vi "Gather Test Data - Heatup Test.vi"(0 "Agilent Scan List":string="101,102,103,104,105,106,107,108,109,110,111,112,113,114,115,116", 1 "Semiphore":T3, 2 "Equipment":T5={"COM Port"="COM1", "MW100"="MW100", "AG34970"="A-34972A", "Chamber"="WT500"}, 5 "Tank Display Ref":refnum<vi>, 7 "Agilent?":bool=TRUE, 9 "No Serial?":bool, 11 "error in (no error)":errorcluster, 12 "Voltage":dbl=240.0) -> (4 "Tc Tree":dbl[](array[numeric]) format="%.4f", 6 "Output Data":string[][](array[string]), 8 "POWER":T1, 10 "PowerData":T2={"Voltage"=236.2, "Current"=17.749, "Power"=4192.0, "WattHours"=0.0}, 15 "error out":errorcluster={"status"=TRUE, "code"=-1073807346, "source"="VISA Read in Gather Test Data.vi"})   [LabVIEW 2009]
uses:
  EquipReferences.ctl
  HEWH Tank Indicator.ctl
  PowerData.ctl
  PowerElements.ctl
panel:
  out "Flow(GPM)":dbl
  out "Gallons":dbl
  out "Output Data View":string[][](array[string])
  out "Tambient":dbl
  out "34970 Data":string[](array[string])=["32.000000E+0"]
  out "WT500 Data":string[](array[string])=["0.000000E+0", "0.000000E+0", "0.000000E+0", "0.000000E+0"]
  out "Local Tank Display":T4 {"TC6" format="%.2g"; "TIN" format="%.2g"; "TOUT" format="%.2g"; "Mean" format="%.2f"; "Std Dev" format="%.2f"; "TC5" format="%.2g"; "TC4" format="%.2g"; "TC3" format="%.2g"; "TC2" format="%.2g"; "TC1" format="%.2g"}
  out "MW100 Data":string[](array[string])=["0.000000E+0", "0.000000E+0"]
  out "Serial Data":string
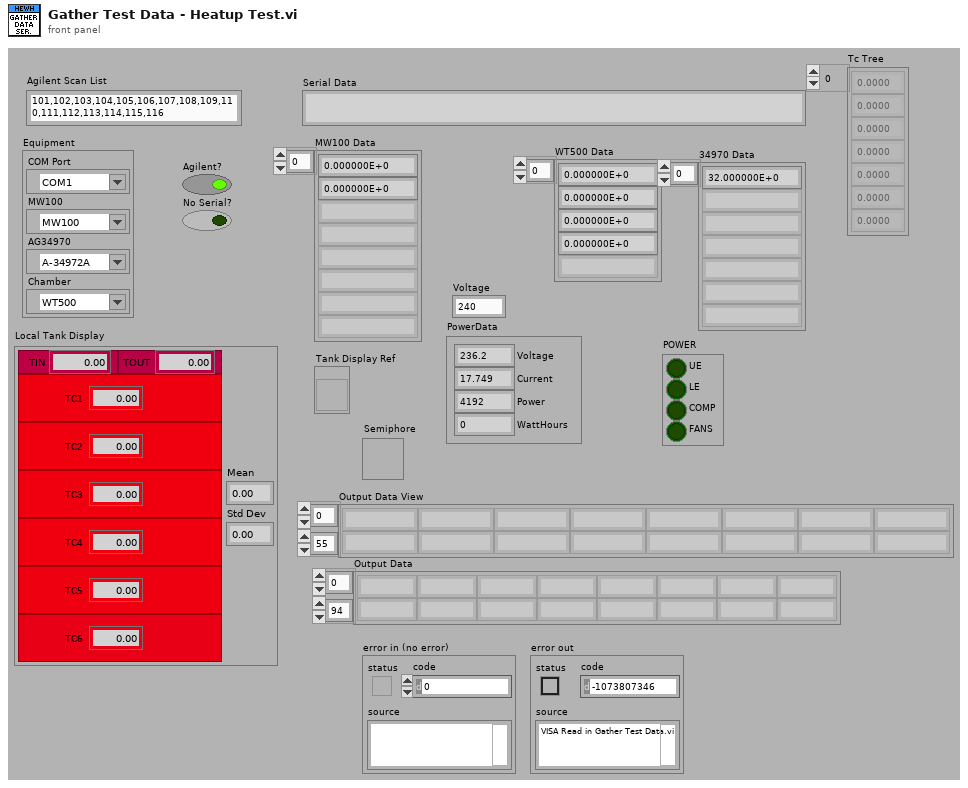
[diagram p1: front panel]
types:
  T1 = typedef "PowerElements.ctl" = cluster{"UE":bool, "LE":bool, "COMP":bool, "FANS":bool}
  T2 = typedef "PowerData.ctl" = cluster{"Voltage":dbl, "Current":dbl, "Power":dbl, "WattHours":dbl}
  T3 = typedef "Semaphore RefNum" = refnum<k1>
  T4 = typedef "HEWH Tank Indicator.ctl" = cluster{"TC1-D":bool, "TC2-D":bool, "TC3-D":bool, "TC4-D":bool, "TC5-D":bool, "RTD_IN":bool, "RTDOUT":bool, "TC1":dbl, "TC2":dbl, "TC3":dbl, "TC4":dbl, "TC5":dbl, "TIN":dbl, "TOUT":dbl, "Std Dev":dbl, "Mean":dbl, "TC6-D":bool, "TC6":dbl}
  T5 = typedef "EquipReferences.ctl" = cluster{"COM Port":refnum<visa-resource-name>, "MW100":refnum<visa-resource-name>, "AG34970":refnum<visa-resource-name>, "Chamber":refnum<visa-resource-name>}
  T6 = typedef "PowerClassification.ctl" = cluster{"Off":bool, "On":bool, "Fans":bool, "Compressor":bool, "Heat Elem.":bool, "Fault-OverPwr":bool}
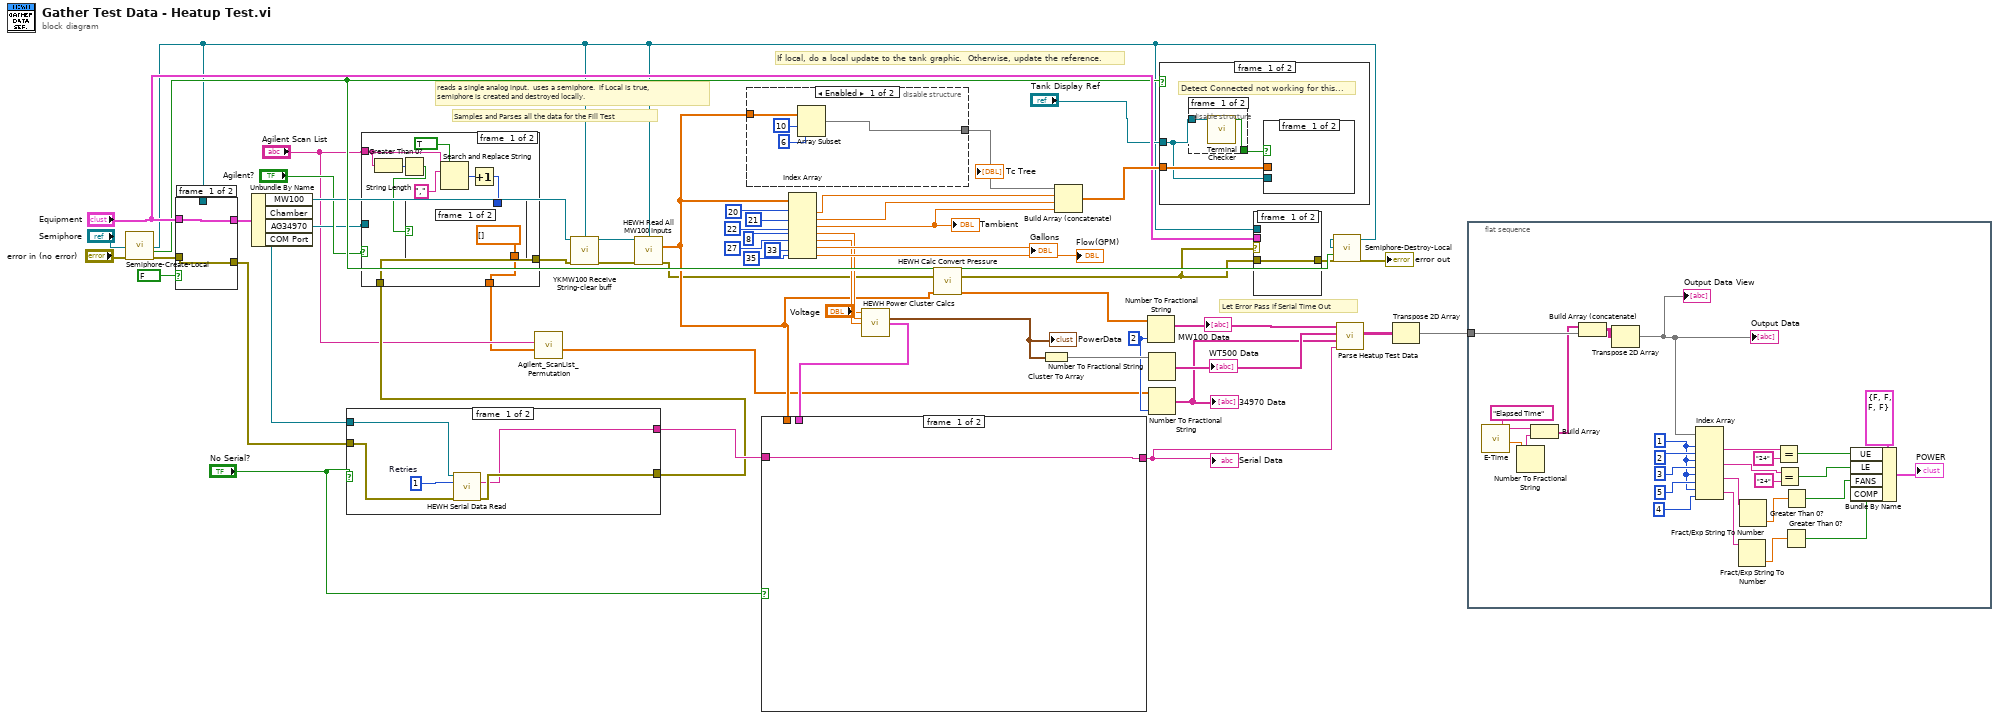
[diagram p0: block diagram]
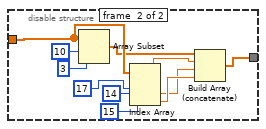
[diagram p2: hidden frame]
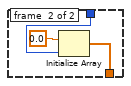
[diagram p3: hidden frame]
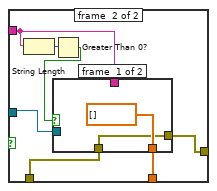
[diagram p4: hidden frame]
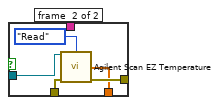
[diagram p5: hidden frame]
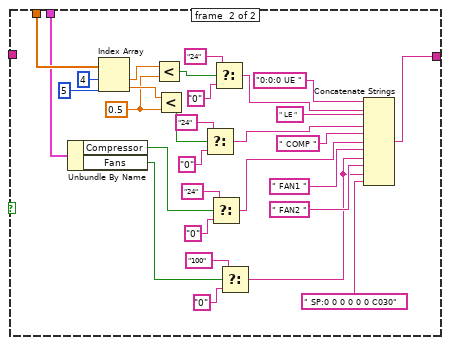
[diagram p6: hidden frame]
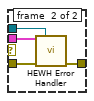
[diagram p7: hidden frame]
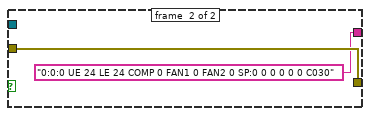
[diagram p8: hidden frame]
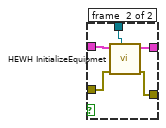
[diagram p9: hidden frame]
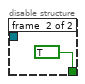
[diagram p10: hidden frame]
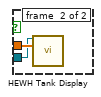
[diagram p11: hidden frame]
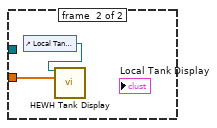
[diagram p12: hidden frame]
diagram:
  w7 = i16 2 ("precision (6)")
  # "Let Error Pass if Serial Time Out"
  # "reads a single analog input.  uses a semiphore.  if Local is true, \nsemiphore is created and destroyed locally."
  # "If local, do a local update to the tank graphic.  Otherwise, update the reference."
  # "Samples and Parses all the data for the Fill Test"
  n1 = call "Semiphore-Create-Local.vi"("Semiphore"="Semiphore", "error in (no error)"="error in (no error)") -> ("semaphore"=w13:T3, "Local?"=w40:bool, "error out"=w46:errorcluster)  [unwired: 15 in]
  n2 = case shown="True" FALSE ("No Serial?") {
    tunnel: [w57 w61] -> w47
    tunnel: "Equipment" -> [w57 w62]
    tunnel: w46 -> [w56 w60]
    tunnel: [w56 w59] -> w45
    tunnel: w13 -> [_ w58]
    frame #0 {
    }
    frame #1 {
      n3 = call "HEWH InitializeEquipmet.vi"("Semiphore"=w58, "Error In"=w60, "Equipment"=w62) -> ("Error Out"=w59:errorcluster, "Equipment Out"=w61:T5)  [unwired: 5 in, 2 out]
    }
  }
  n4 = Unbundle By Name(w47) -> ("MW100"=w36:refnum<visa-resource-name>, "AG34970"=w10:refnum<visa-resource-name>, "COM Port"=w50:refnum<visa-resource-name>)  [unwired: 1 out]
  n5 = case shown="False" "No Serial?" {
    tunnel: w50 -> [w65 _]
    tunnel: [w67 w69] -> w9
    tunnel: w45 -> [w64 w69]
    tunnel: [w66 "0:0:0 UE 24 LE 24 COMP 0 FAN1 0 FAN2 0 SP:0 0 0 0 0 0 C030" ("trimmed string")] -> w14
    frame #0 {
      w63 = 1  # Retries
      n6 = call "HEWH Serial Data Read.vi"("Serial Port Ref"=w65, "Retries"=w63, "error in (no error)"=w64) -> ("Read String"=w66:string, "error out"=w67:errorcluster)  [unwired: 11 in]
    }
    frame #1 {
    }
  }
  n7 = case shown="True" "Agilent?" {
    tunnel: [w71 w87] -> w5
    tunnel: w10 -> [_ w85]
    tunnel: "Agilent Scan List" -> [w75 w86]
    tunnel: w9 -> [w78 w84]
    tunnel: [w78 w83] -> w8
    frame #0 {
      n8 = String Length(string=w75) -> (length=w74:i32)
      n9 = Greater Than 0?(x=w74) -> (x > 0?=w73:bool)
      n10 = Search and Replace String(replace all?=TRUE ("ignore case? (F)"), input string=w75, search string=",") -> (number of replacements=w76:i32)  [unwired: 5 in, 3 out]
      n11 = Increment(x=w76) -> (x+1=w72:i32)
      n12 = case shown="True" w73 {
        tunnel: w72 -> [_ w81]
        tunnel: [dbl[] [] w80] -> w71
        frame #0 {
        }
        frame #1 {
          n13 = Initialize Array(0.0, w81) -> (w80:dbl[])
        }
      }
    }
    frame #1 {
      n14 = String Length(string=w86) -> (length=w89:i32)
      n15 = Greater Than 0?(x=w89) -> (x > 0?=w88:bool)
      n16 = case shown="True" w88 {
        tunnel: [dbl[] [] w93] -> w87
        tunnel: w86 -> [_ _]
        tunnel: w85 -> [_ w96]
        tunnel: w84 -> [w90 w95]
        tunnel: [w90 w94] -> w83
        frame #0 {
        }
        frame #1 {
          n17 = call "Agilent Scan EZ Temperature.vi"("VISA Resource Name"=w96, "Control"=enum16{"Initialize", "Read", "Experiment"}."Read", "error in (no error)"=w95) -> ("Output Array"=w93:dbl[], "error out"=w94:errorcluster)  [unwired: 9 in, 2 out]
        }
      }
    }
  }
  n18 = call "Agilent_ScanList_Permutation.vi"("Input Data Array"=w5, "Agilent Scan List"="Agilent Scan List") -> ("Output Data Permutation"=w1:dbl[])  [unwired: 9 in]
  n19 = call "YKMW100 Receive String-clear buff.vi"("VISA session"=w36, "Semiphore"=w13, "error in (no error)"=w8) -> ("dup VISA session"=w35:refnum<visa-resource-name>, "error out"=w34:errorcluster)  [unwired: 10 in, 1 out]
  n20 = call "HEWH Read All MW100 Inputs.vi"("MW100"=w35, "Semiphore"=w13, "Error In"=w34) -> ("All Data"=w4:dbl[], "error out"=w2:errorcluster)  [unwired: 10 in, 1 out]
  n21 = disable-structure shown="Enabled" {
    disable-tunnel: [w98 w105] -> w33
    disable-tunnel: w4 -> [w97 w109]
    frame #0 {
      n22 = Array Subset(array=w97, index=10, length=6) -> (w98:dbl[])
    }
    frame #1 {
      n23 = Array Subset(array=w109, index=10, length=3) -> (w101:dbl[])
      n24 = Index Array(array=w109, index #1=17 ("index"), index #2=14 ("index"), index #3=15 ("index")) -> (element #1=w102:dbl, element #2=w103:dbl, element #3=w104:dbl)
      n25 = Build Array (concatenate)(w101, w102, w103, w104) -> (w105:dbl[])
    }
  }
  "Tc Tree" <- w33
  n26 = Index Array(array=w4, index #1=20 ("index"), index #2=21 ("index"), index #3=22 ("index"), index #4=8 ("index"), index #5=27 ("index"), index #6=33 ("index"), index #7=35 ("index")) -> (element #1=w31:dbl, element #2=w29:dbl, element #3=w27:dbl, element #4=w20:dbl, element #5=w19:dbl, element #6=→"Gallons":dbl, element #7=→"Flow(GPM)":dbl)
  "Tambient" <- w27
  n27 = call "HEWH Power Cluster Calcs.vi"("Voltage"="Voltage", "Watts"=w20, "WattHours"=w19) -> ("PowerData"=w18:T2, "PowerClass"=w16:T6)  [unwired: 11 in]
  "PowerData" <- w18
  n28 = case shown="True" "No Serial?" {
    tunnel: w4 -> [_ w142]
    tunnel: w16 -> [_ w136]
    tunnel: [w112 w119] -> w15
    tunnel: w14 -> [w112 _]
    frame #0 {
    }
    frame #1 {
      w137 = 0.5 ("y")
      n29 = Unbundle By Name(w136) -> ("Compressor"=w120:bool, "Fans"=w116:bool)
      n30 = Index Array(array=w142, index #1=4 ("index"), index #2=5 ("index")) -> (element #1=w139:dbl, element #2=w138:dbl)
      n31 = Less?(x=w139, y=w137) -> (x < y?=w122:bool)
      n32 = Less?(x=w138, y=w137) -> (x < y?=w121:bool)
      n33 = Select(t="24" ("trimmed string"), s=w121, f="0" ("trimmed string")) -> (s? t:f=w134:string)
      n34 = Select(t="24" ("trimmed string"), s=w120, f="0" ("trimmed string")) -> (s? t:f=w135:string)
      n35 = Select(t="24" ("trimmed string"), s=w122, f="0" ("trimmed string")) -> (s? t:f=w133:string)
      n36 = Select(t="100" ("trimmed string"), s=w116, f="0" ("trimmed string")) -> (s? t:f=w114:string)
      n37 = Concatenate Strings("0:0:0 UE " ("trimmed string"), w133, " LE " ("trimmed string"), w134, " COMP " ("trimmed string"), w135, " FAN1 " ("trimmed string"), w114, " FAN2 " ("trimmed string"), w114, " SP:0 0 0 0 0 0 C030" ("trimmed string")) -> (w119:string)
    }
  }
  "Serial Data" <- w15
  n38 = call "HEWH Calc Convert Pressure.vi"("All Data"=w4) -> ("output array"=w3:dbl[])  [unwired: 10 in]
  n39 = Cluster To Array(cluster=w18) -> (array=w54:dbl[])
  n40 = Build Array (concatenate)(w33, w31, w29, w27) -> (w51:dbl[])
  n41 = Number To Fractional String(number=w3, precision (6)=w7) -> (F-format string=w55:string[])  [unwired: 2 in]
  "MW100 Data" <- w55
  n42 = Number To Fractional String(number=w54) -> (F-format string=w53:string[])  [unwired: 3 in]
  "WT500 Data" <- w53
  n43 = Number To Fractional String(number=w1, precision (6)=w7) -> (F-format string=w52:string[])  [unwired: 2 in]
  "34970 Data" <- w52
  n44 = case shown="True" w40 {
    tunnel: w51 -> [w145 w152]
    tunnel: "Tank Display Ref" -> [w143 _]
    frame #0 {
      # "Detect Connected not working for this..."
      n45 = disable-structure shown="Enabled" {
        disable-tunnel: [w147 TRUE ("is connected?")] -> w144
        disable-tunnel: w143 -> [w146 _]
        frame #0 {
          n46 = call "Terminal Checker.vi"("control reference"=w146) -> ("is connected?"=w147:bool)  [unwired: 9 in, 1 out]
        }
        frame #1 {
        }
      }
      n47 = case shown="True" w144 {
        tunnel: w145 -> [_ w150]
        tunnel: w143 -> [_ w149]
        frame #0 {
        }
        frame #1 {
          n48 = call "HEWH Tank Display.vi"("Local Tank Display"=w149, "T1-T6.Tin,Tout"=w150) -> ()  [unwired: 13 in, 1 out]
        }
      }
    }
    frame #1 {
      n49 = control-ref of="Local Tank Display"() -> (w151:refnum<vi>)
      n50 = call "HEWH Tank Display.vi"("Local Tank Display"=w151, "T1-T6.Tin,Tout"=w152) -> ()  [unwired: 13 in, 1 out]
    }
  }
  n51 = case shown="Error" w2 {
    tunnel: "Equipment" -> [_ w157]
    tunnel: [w153 w156] -> w39
    tunnel: w13 -> [_ w155]
    tunnel: w2 -> [w153 w154]
    frame #0 {
    }
    frame #1 {
      n52 = call "HEWH Error Handler.vi"("Equipment"=w157, "MW100 Semiphore"=w155, "error in (no error)"=w154) -> ("Error Out (no error)"=w156:errorcluster)  [unwired: 12 in]
    }
  }
  n53 = call "Semiphore-Destroy-Local.vi"("Semiphore"=w13, "Local?"=w40, "error in (no error)"=w39) -> ("error out"=→"error out":errorcluster)  [unwired: 16 in]
  n54 = call "Parse Heatup Test Data.vi"("Serial Data"=w15, "34970 Data"=w52, "Power Data"=w53, "MW100 Data"=w55) -> ("Output Data"=w44:string[][])  [unwired: 7 in]
  n55 = Transpose 2D Array(2D array=w44) -> (transposed array=w43:string[][])
  n56 = flat-sequence {
    tunnel: w43 -> [w183]
    frame #0 {
      w160 = 1 ("index (row)")
      n57 = call "E-Time.vi"() -> ("Elapsed Time (sec)"=w166:dbl)  [unwired: 9 in, 2 out]
      n58 = Number To Fractional String(number=w166) -> (F-format string=w179:string)  [unwired: 3 in]
      n59 = Build Array("Elapsed Time" ("Serial Data 2"), w179) -> (w181:string[])
      n60 = Build Array (concatenate)(w181, w183) -> (w180:string[][])
      n61 = Transpose 2D Array(2D array=w180) -> (transposed array=w165:string[][])
      "Output Data" <- w165
      "Output Data View" <- w165
      n62 = Index Array(array=w165, index (row) #1=w160, index (col) #1=2 ("disabled index (col)"), index (row) #2=w160, index (col) #2=3 ("disabled index (col)"), index (row) #3=w160, index (col) #3=5 ("disabled index (col)"), index (row) #4=w160, index (col) #4=4 ("disabled index (col)")) -> (element #1=w175:string, element #2=w173:string, element #3=w164:string, element #4=w158:string)
      n63 = Fract/Exp String To Number(string=w158) -> (number=w162:dbl)  [unwired: 3 in, 1 out]
      n64 = Fract/Exp String To Number(string=w164) -> (number=w163:dbl)  [unwired: 3 in, 1 out]
      n65 = Equal?(x=w175, y="24") -> (x = y?=w169:bool)
      n66 = Equal?(x=w173, y="24") -> (x = y?=w168:bool)
      n67 = Greater Than 0?(x=w162) -> (x > 0?=w161:bool)
      n68 = Greater Than 0?(x=w163) -> (x > 0?=w167:bool)
      n69 = Bundle By Name(cluster=T1 {"UE"=FALSE, "LE"=FALSE, "COMP"=FALSE, "FANS"=FALSE} ("POWER"), "UE"=w169, "LE"=w168, "FANS"=w167, "COMP"=w161) -> (→"POWER":T1)
    }
  }
